vi "Close.vi"(8 "error in":errorcluster, 11 "MouseEventArgs in":refnum<class "MouseEventArgs.lvclass">) -> (0 "error out":errorcluster, 3 "MouseEventArgs out":refnum<class "MouseEventArgs.lvclass">)   [LabVIEW 2024, in "SourceGrid.lvlib" / "MouseEventArgs.lvclass"]
uses:
  MouseEventArgs.lvclass
  MouseEventArgs.lvclass/MouseEventArgs.ctl
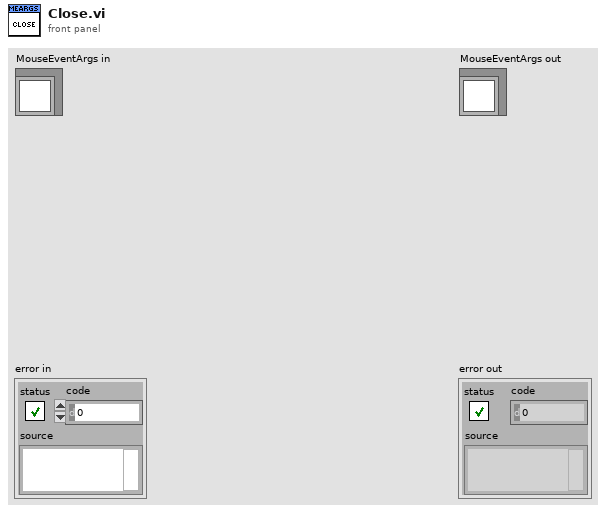
[diagram p1: front panel]
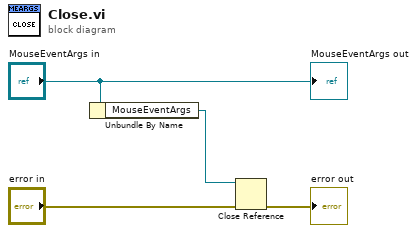
[diagram p0: block diagram]
diagram:
  n1 = Unbundle By Name("MouseEventArgs in") -> ("MouseEventArgs"=w1:refnum<k24>)
  n2 = Close Reference(reference=w1, error in (no error)="error in") -> (error out=→"error out":errorcluster)
  "MouseEventArgs out" <- "MouseEventArgs in"
